vi "NI VeriStand - Get Asynchronous Driver VI Timed Loop Name.vi"(8 "error in (no error)":errorcluster, 11 "Device Ref in":T1 format="%.0x") -> (0 "error out":errorcluster, 2 "Device Timed Loop Name":string, 3 "Device Ref out":T1 format="%.0x")   [LabVIEW 2020, in "Custom Device API.lvlib"]
doc: "Returns the name of the Timed Loop that an asynchronous custom device uses. The VeriStand Engine synchronizes the start of this Timed Loop with the other system Timed Loops. Use the Timed Loop name this VI returns to ensure this synchronization occurs successfully."
uses:
  <vilib>/NI VeriStand/Custom Device API/Custom Device API.lvlib
  <vilib>/NI VeriStand/Custom Device API/Custom Device Item Ref.ctl
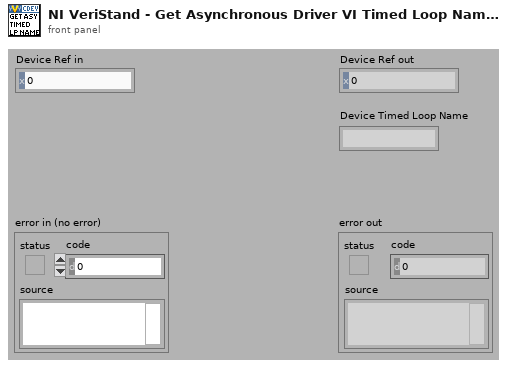
[diagram p1: front panel]
types:
  T1 = typedef "Custom Device API.lvlib/Custom Device Item Ref.ctl" = u64
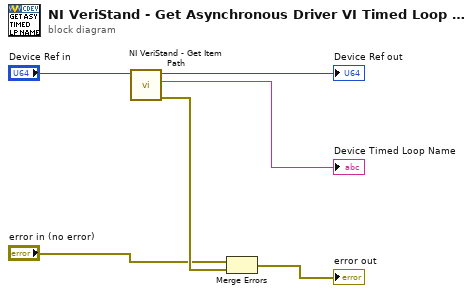
[diagram p0: block diagram]
diagram:
  n1 = call <vilib>:"NI VeriStand - Get Item Path.vi"("Item Ref in"="Device Ref in") -> ("error out"=w3:errorcluster, "Path"=→"Device Timed Loop Name":string, "Item Ref out"=→"Device Ref out":T1)  [unwired: 1 in, 7 out]
  n2 = Merge Errors("error in (no error)", w3) -> (→"error out":errorcluster)
